vi "read keypad.vi"(7 "scan interval [ms]":u32=10, 8 "error in (no error)":errorcluster, 11 "keypad ref":T1={"column drivers"={"myRIO Reference"={"myRIO Model"=enum."Unknown", "myRIO Hardware Reference"={"Generic FPGA Reference"=refnum, "Allow multiple opens"=FALSE}}, "DIO Channels List"=[]}, "row drivers"={"myRIO Reference"={"myRIO Model"=enum."Unknown", "myRIO Hardware Reference"={"Generic FPGA Reference"=refnum, "Allow multiple opens"=FALSE}}, "DIO Channels List"=[]}, "pull downs"=FALSE, "timeout [ms]"=4294967295}) -> (0 "error out":errorcluster, 1 "timed out":bool, 2 "keypad code":i32, 3 "keypad ref out":T1={"column drivers"={"myRIO Reference"={"myRIO Model"=enum."Unknown", "myRIO Hardware Reference"={"Generic FPGA Reference"=refnum, "Allow multiple opens"=FALSE}}, "DIO Channels List"=[]}, "row drivers"={"myRIO Reference"={"myRIO Model"=enum."Unknown", "myRIO Hardware Reference"={"Generic FPGA Reference"=refnum, "Allow multiple opens"=FALSE}}, "DIO Channels List"=[]}, "pull downs"=FALSE, "timeout [ms]"=4294967295})   [LabVIEW 2013]
uses:
  keypad references.ctl
  <vilib>/myRIO/Instrument Drivers/Onboard IO/DIO/typedefs/DIO Reference.ctl
  <vilib>/myRIO/Common/Instrument Driver Framework/Utilities/typedefs/myRIO Generic Hardware Reference.ctl
  <vilib>/myRIO/Common/Instrument Driver Framework/Utilities/typedefs/Hardware Version Enum.ctl
  <vilib>/myRIO/Common/Instrument Driver Framework/Utilities/typedefs/myRIO v1.0 Reference.ctl
  <vilib>/myRIO/Common/Instrument Driver Framework/Utilities/typedefs/Generic FPGA Reference.ctl
  <vilib>/myRIO/Common/Instrument Driver Framework/myRIO v1.0/DIO/typedefs/DIO Channels List.ctl
  <vilib>/myRIO/Common/Instrument Driver Framework/myRIO v1.0/DIO/typedefs/DIO Channels Enum.ctl
  <vilib>/myRIO/Instrument Drivers/Onboard IO/DIO/DIO.lvlib
panel:
  # "read keypad"
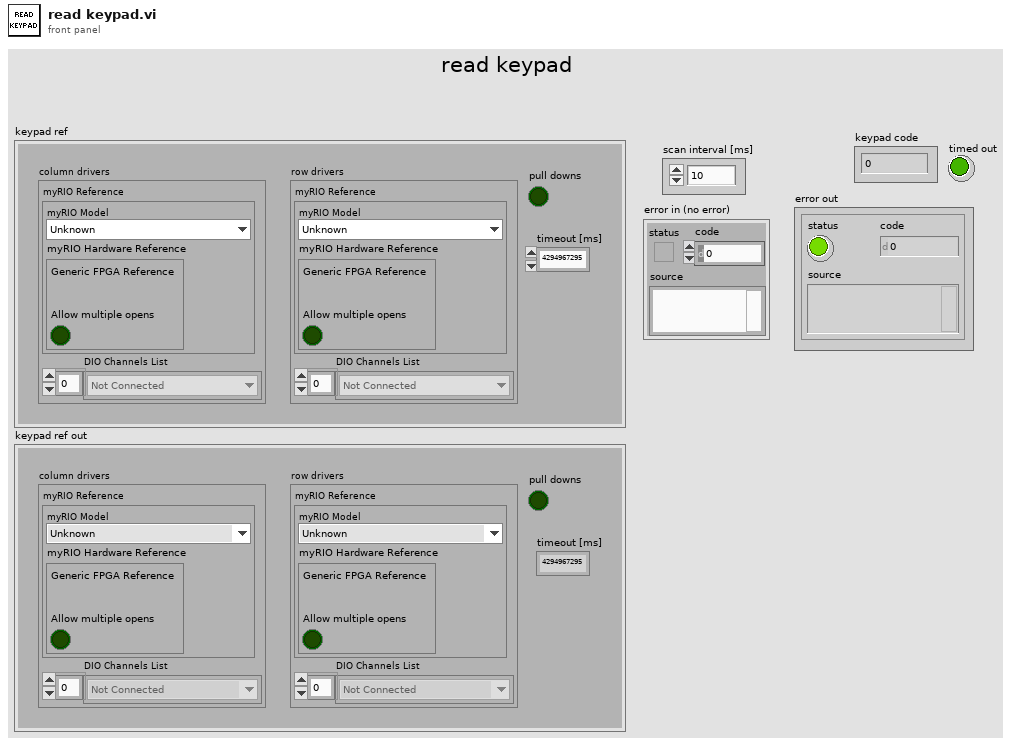
[diagram p1: front panel]
types:
  T1 = typedef "keypad references.ctl" = cluster{"column drivers":T2, "row drivers":T2, "pull downs":bool, "timeout [ms]":u32}
  T2 = typedef "DIO.lvlib/DIO Reference.ctl" = cluster{"myRIO Reference":T3, "DIO Channels List":T7}
  T3 = typedef "myRIO Generic Hardware Reference.ctl" = cluster{"myRIO Model":T4, "myRIO Hardware Reference":T5}
  T4 = typedef "Hardware Version Enum.ctl" = enum16{"Unknown", "myRIO-1900", "myRIO-1950"}
  T5 = typedef "myRIO v1.0 Reference.ctl" = cluster{"Generic FPGA Reference":T6, "Allow multiple opens":bool}
  T6 = typedef "Generic FPGA Reference.ctl" = refnum<k20>
  T7 = typedef "DIO Channels List.ctl" = T8[]
  T8 = typedef "DIO Channels Enum.ctl" = enum16{"Not Connected", "C/DIO0", "C/DIO1", "C/DIO2", "C/DIO3", "C/DIO4", "C/DIO5", "C/DIO6", "C/DIO7", "A/DIO0", "A/DIO1", "A/DIO2", "A/DIO3", "A/DIO4", "A/DIO5", "A/DIO6", "A/DIO7", "A/DIO8", "A/DIO9", "A/DIO10", "A/DIO11", "A/DIO12", "A/DIO13", "A/DIO14", "A/DIO15", "B/DIO0", "B/DIO1", "B/DIO2", "B/DIO3", "B/DIO4", "B/DIO5", "B/DIO6", "B/DIO7", "B/DIO8", "B/DIO9", "B/DIO10", "B/DIO11", "B/DIO12", "B/DIO13", "B/DIO14", "B/DIO15", "LED0", "LED1", "LED2", "LED3", "Button0"}
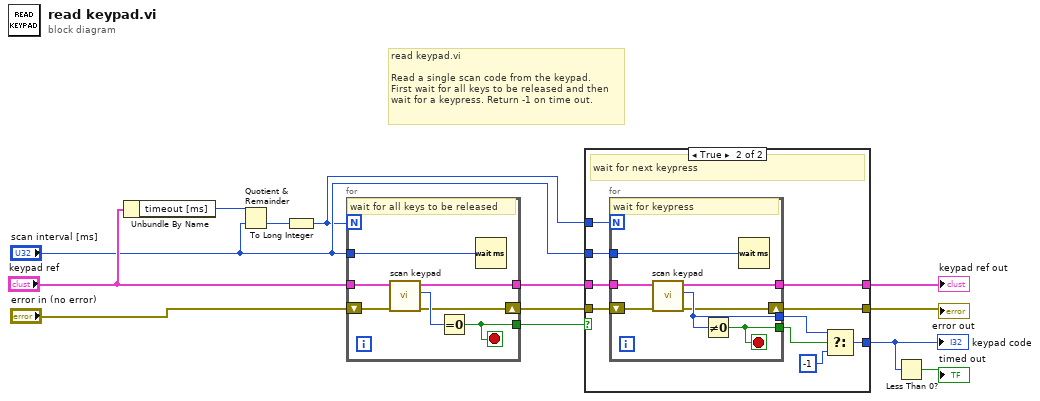
[diagram p0: block diagram]
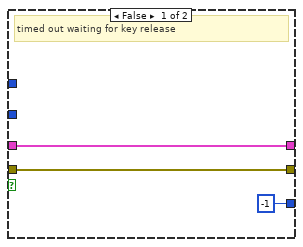
[diagram p2: hidden frame]
diagram:
  # "read keypad.vi\n\nRead a single scan code from the keypad.\nFirst wait for all keys to be released and then\nwait for a keypress. Return -1 on time out."
  n1 = Unbundle By Name("keypad ref") -> ("timeout [ms]"=w12:u32)
  n2 = Quotient & Remainder(x=w12, y="scan interval [ms]") -> (floor(x/y)=w2:u32)  [unwired: 1 out]
  n3 = To Long Integer(number=w2) -> (32bit integer=w1:i32)
  n4 = for {
    N: w1 -> [_]
    tunnel: "keypad ref" -> [w20]
    tunnel: "scan interval [ms]" -> [w19]
    tunnel: [w18] -> w9
    tunnel: [w16] -> w8
    shift-right: [w14] -> w6
    shift-left: "error in (no error)" -> [w15]
    stop <- w16 stop-if-true
    # "wait for all keys to be released"
    n5 = call "scan keypad.vi"("error in (no error)"=w15, "keypad ref"=w20) -> ("error out"=w14:errorcluster, "keypad code"=w17:i32, "keypad ref out"=w18:T1)  [unwired: 7 in]
    n6 = Equal To 0?(x=w17) -> (x = 0?=w16:bool)
    n7 = Wait (ms)(milliseconds to wait=w19) -> ()  [unwired: 1 out]
  }
  n8 = case shown="True" w8 {
    tunnel: [w22 w33] -> w11
    tunnel: "scan interval [ms]" -> [_ w32]
    tunnel: w1 -> [_ w31]
    tunnel: w9 -> [w22 w30]
    tunnel: [-1 w28] -> w4
    tunnel: w6 -> [w21 w25]
    tunnel: [w21 w24] -> w5
    frame False {
      # "timed out waiting for key release"
    }
    frame True {
      # "wait for next keypress"
      n9 = for {
        N: w31 -> [_]
        tunnel: w30 -> [w40]
        tunnel: w32 -> [w39]
        tunnel: [w37] -> w29
        tunnel: [w38] -> w33
        tunnel: [w36] -> w27
        shift-right: [w34] -> w24
        shift-left: w25 -> [w35]
        stop <- w36 stop-if-true
        # "wait for keypress"
        n10 = call "scan keypad.vi"("error in (no error)"=w35, "keypad ref"=w40) -> ("error out"=w34:errorcluster, "keypad code"=w37:i32, "keypad ref out"=w38:T1)  [unwired: 7 in]
        n11 = Not Equal To 0?(x=w37) -> (x != 0?=w36:bool)
        n12 = Wait (ms)(milliseconds to wait=w39) -> ()  [unwired: 1 out]
      }
      n13 = Select(t=w29, s=w27, f=-1) -> (s? t:f=w28:i32)
    }
  }
  "keypad code" <- w4
  "keypad ref out" <- w11
  "error out" <- w5
  n14 = Less Than 0?(x=w4) -> (x < 0?=→"timed out":bool)
